vi "Init.vi"(8 "error in (no error)":errorcluster, 11 "Data in":refnum<class "Remap Bus.lvclass">) -> (0 "error out":errorcluster, 3 "Data out":refnum<class "Remap Bus.lvclass">)   [LabVIEW 2021, in "Remap Bus.lvclass"]
doc: "Abstract Data Classes 2.1.1.12\nTim Streeter - TSA\nCopyright (c) 2024, TSA"
uses:
  Remap Bus.lvclass
  C:/Users/Tim/Documents/GitHub/Omni-Bus/Source/Omni-Bus/Bus Access/Bus_Access.lvclass
  Remap Bus.lvclass/Remap Bus.ctl
  Omni-Bus/Bus Access/Bus_Access.lvclass/Bus_Access.ctl
  Omni-Bus/Bus Access/Properties/Read Tags.vi
  Omni-Bus/Bus Access/Properties/Read Values.vi
  Properties/Read Buses.vi
  Properties/Read Map.vi
  Properties/Read Keep Original.vi
  Properties/Write Buses.vi
  Omni-Bus/Bus Access/Properties/Write Tags.vi
  Omni-Bus/Bus Access/Properties/Write Values.vi
  Omni-Bus/Bus Access/Bus_Access.lvclass
  <vilib>/TSA/Abstract Data Classes/Abs_Types/Type/Abs_Type.lvclass
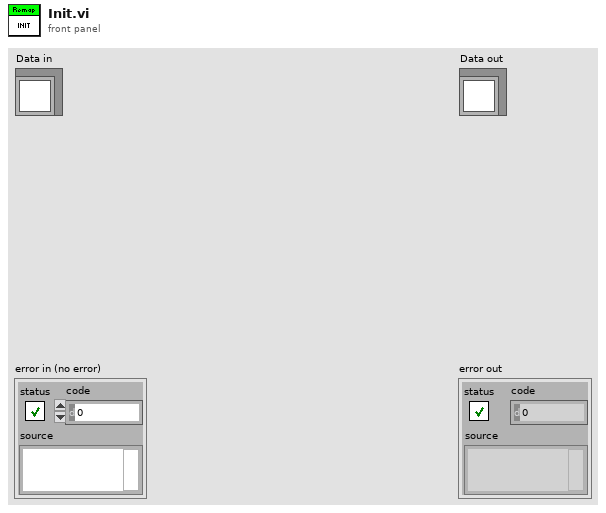
[diagram p1: front panel]
types:
  T1 = typedef "Remap Bus.lvclass/Remap Type.ctl" = map{string, string}
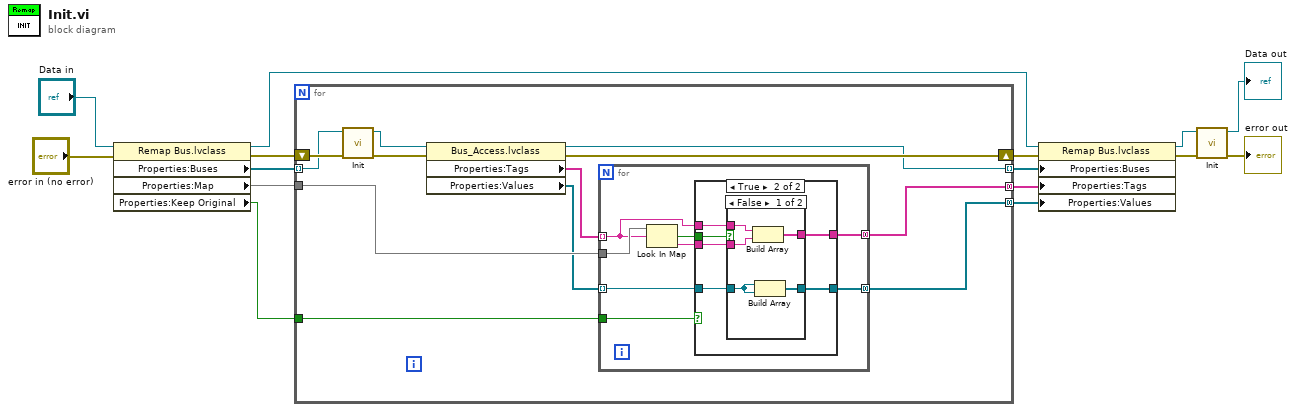
[diagram p0: block diagram]
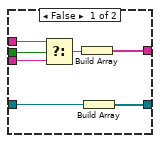
[diagram p2: hidden frame]
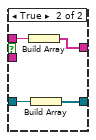
[diagram p3: hidden frame]
diagram:
  n1 = property class="Remap Bus.lvclass"(reference="Data in", error in="error in (no error)") -> (reference out=w8:refnum<class "Remap Bus.lvclass">, error out=w12:errorcluster, "Properties:Buses"=w13:refnum<class "Bus_Access.lvclass">[], "Properties:Map"=w11:T1, "Properties:Keep Original"=w5:bool)
  n2 = for {
    tunnel: w13 -> [w24] mode=indexing
    shift-right: [w21] -> w10
    shift-left: w12 -> [w25]
    tunnel: w11 -> [w27]
    tunnel: [w20] -> w9 mode=indexing
    tunnel: [w19] -> w7 mode=concatenating
    tunnel: [w17] -> w6 mode=concatenating
    tunnel: w5 -> [w16]
    n3 = call-dynamic "Init.vi"("error in (no error)"=w25, "Data in"=w24) -> ("error out"=w23:errorcluster, "Data out"=w22:refnum<class "Bus_Access.lvclass">)  [unwired: 8 in]
    n4 = property class="Bus_Access.lvclass"(reference=w22, error in=w23) -> (reference out=w20:refnum<class "Bus_Access.lvclass">, error out=w21:errorcluster, "Properties:Tags"=w26:string[], "Properties:Values"=w18:refnum<class "Abs_Type.lvclass">[])
    n5 = for {
      tunnel: w27 -> [w35]
      tunnel: w26 -> [w32] mode=indexing
      tunnel: [w30] -> w19 mode=concatenating
      tunnel: w18 -> [w31] mode=indexing
      tunnel: [w29] -> w17 mode=concatenating
      tunnel: w16 -> [w28]
      n6 = Look In Map(map=w35, key=w32) -> (key not found?=w33:bool, value=w34:string)  [unwired: 1 in]
      n7 = case shown="True" w28 {
        tunnel: w34 -> [w42 w47]
        tunnel: w33 -> [w41 w48]
        tunnel: w32 -> [w40 w46]
        tunnel: [w36 w45] -> w30
        tunnel: w31 -> [w38 w44]
        tunnel: [w37 w43] -> w29
        frame False {
          n8 = Select(t=w40, s=w41, f=w42) -> (s? t:f=w39:string)
          n9 = Build Array(w39) -> (w36:string[])
          n10 = Build Array(w38) -> (w37:refnum<class "Abs_Type.lvclass">[])
        }
        frame True {
          n11 = case shown="False" w48 {
            tunnel: w47 -> [w52 _]
            tunnel: w46 -> [w53 w57]
            tunnel: [w51 w56] -> w45
            tunnel: w44 -> [w50 w55]
            tunnel: [w49 w54] -> w43
            frame False {
              n12 = Build Array(w53, w52) -> (w51:string[])
              n13 = Build Array(w50, w50) -> (w49:refnum<class "Abs_Type.lvclass">[])
            }
            frame True {
              n14 = Build Array(w57) -> (w56:string[])
              n15 = Build Array(w55) -> (w54:refnum<class "Abs_Type.lvclass">[])
            }
          }
        }
      }
    }
  }
  n16 = property class="Remap Bus.lvclass"(reference=w8, error in=w10, "Properties:Buses"=w9, "Properties:Tags"=w7, "Properties:Values"=w6) -> (reference out=w2:refnum<class "Remap Bus.lvclass">, error out=w4:errorcluster)
  n17 = call-parent "Init.vi"("error in (no error)"=w4, "Data in"=w2) -> ("error out"=→"error out":errorcluster, "Data out"=→"Data out":refnum<class "Remap Bus.lvclass">)  [unwired: 8 in]
